vi "Configure Temperature.vi"(6 "Units (1: Celcius)":i32(ring)=1 items=["Kelvin", "Celcius", "Farenheit"], 8 "error in (no error)":errorcluster, 9 "Resolution (1: 6.5 Digits)":i32(ring)=1 items=["5.5 Digits", "6.5 Digits", "7.5 Digits", "8.5 Digits"], 10 "Probe Identity (Probe1)":string="Probe1", 11 "VISA resource name":refnum<visa-resource-name>) -> (0 "error out":errorcluster, 3 "VISA resource name out":refnum<visa-resource-name>)   [LabVIEW 2011, in "Fluke 8508.lvlib"]
doc: "This VI sets the PRT function for temperature measurement on the instrument for a given probe and also sets the units and resolution of the reading.\n\nNOTE:\nThis VI can be run only if the Probe Identity specified already exists on the instrument or it will return an error. To create a new probe, run the appropriate Configure <conversion type> Conversion VI and then run this VI to set the temperature function."
uses:
  Fluke 8508.lvlib
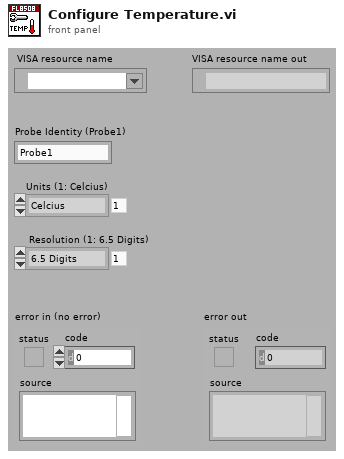
[diagram p1: front panel]
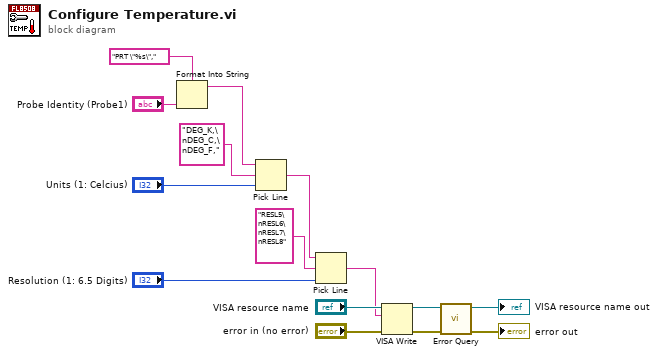
[diagram p0: block diagram]
diagram:
  n1 = Format Into String(format string="PRT \"%s\",", "Probe Identity (Probe1)") -> (resulting string=w8:string)  [unwired: 2 in, 1 out]
  n2 = Pick Line(string ("")=w8, multi-line string="DEG_K,\nDEG_C,\nDEG_F,", line index="Units (1: Celcius)") -> (output string=w7:string)
  n3 = Pick Line(string ("")=w7, multi-line string="RESL5\nRESL6\nRESL7\nRESL8", line index="Resolution (1: 6.5 Digits)") -> (output string=w5:string)
  n4 = VISA Write(VISA resource name="VISA resource name", write buffer=w5, error in (no error)="error in (no error)") -> (VISA resource name out=w4:refnum<visa-resource-name>, error out=w3:errorcluster)  [unwired: 1 out]
  n5 = call "Error Query.vi"("error in (no error)"=w3, "VISA resource name"=w4) -> ("error out"=→"error out":errorcluster, "VISA resource name out"=→"VISA resource name out":refnum<visa-resource-name>)  [unwired: 6 in, 2 out]
